vi "teensySweepFreq.vi"(8 "error in (no error)":errorcluster, 9 "end f, Hz (1385)":i32, 10 "start f, Hz (1355)":i32=1355, 11 "VISA Refnum in":refnum<visa-resource-name>) -> (0 "error out":errorcluster)   [LabVIEW 2011]
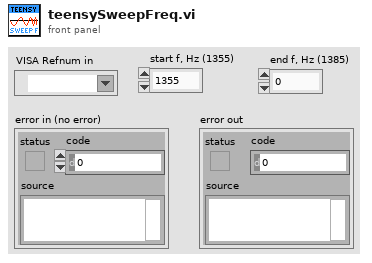
[diagram p1: front panel]
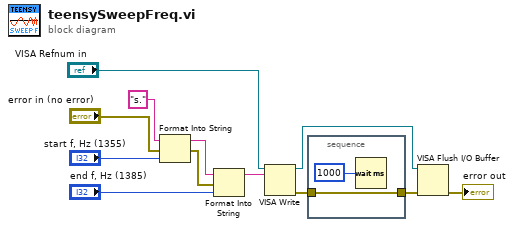
[diagram p0: block diagram]
diagram:
  n1 = Format Into String(initial string="s.", error in="error in (no error)", "start f, Hz (1355)") -> (resulting string=w3:string, error out=w2:errorcluster)  [unwired: 1 in]
  n2 = Format Into String(initial string=w3, error in=w2, "end f, Hz (1385)") -> (resulting string=w1:string)  [unwired: 1 in, 1 out]
  n3 = VISA Write(VISA resource name="VISA Refnum in", write buffer=w1) -> (VISA resource name out=w10:refnum<visa-resource-name>, error out=w9:errorcluster)  [unwired: 1 in, 1 out]
  n4 = stacked-sequence {
    tunnel: w9 -> [w14]
    tunnel: [w14] -> w8
    frame #0 {
      n5 = Wait (ms)(milliseconds to wait=u32 1000) -> ()  [unwired: 1 out]
    }
  }
  n6 = VISA Flush I/O Buffer(VISA resource name=w10, error in (no error)=w8) -> (error out=→"error out":errorcluster)  [unwired: 1 in, 1 out]
